vi "CleanUp.vi"(8 "error in (no error)":errorcluster, 11 "Prueba06 in":refnum<class "Prueba06.lvclass">) -> (0 "error out":errorcluster, 3 "Prueba06 out":refnum<class "Prueba06.lvclass">)   [LabVIEW 2019, in "Prueba06.lvclass"]
uses:
  Prueba06.lvclass
  C:/Users/ivan_/Documents/procal/Pruebas/Prueba/Prueba.lvclass
  Prueba/Prueba.lvclass/Prueba.ctl
  Prueba06.lvclass/Prueba06.ctl
  Base de Datos/SQLiteConnector/SQLiteConnection.lvclass
  Base de Datos/Base de Datos.lvclass
  Prueba/Prueba.lvclass
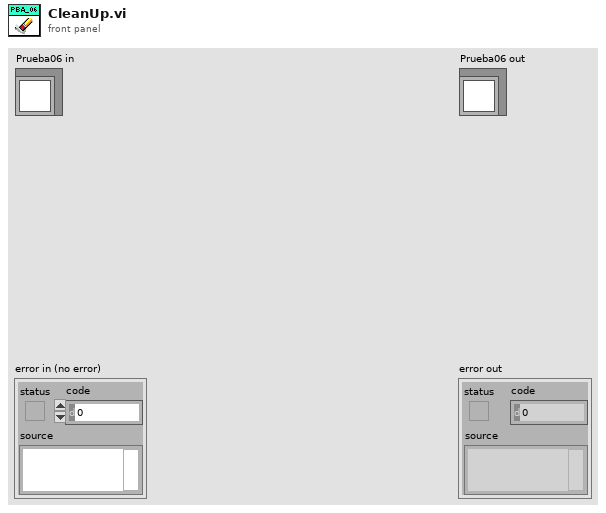
[diagram p1: front panel]
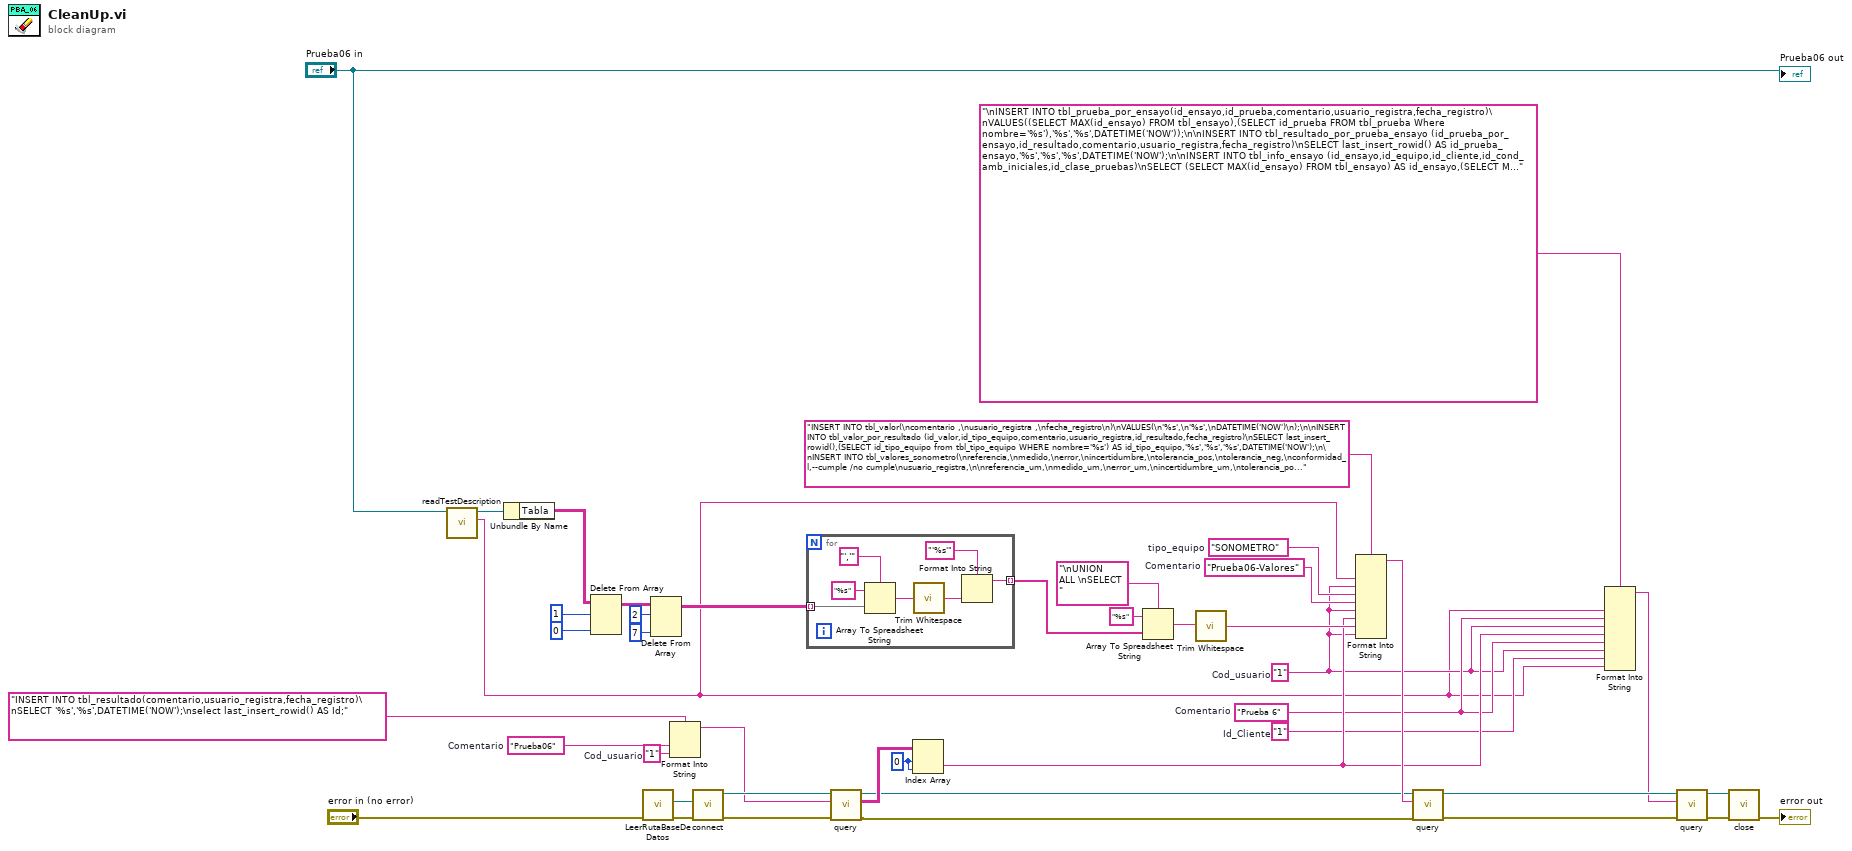
[diagram p0: block diagram]
diagram:
  w15 = "1"  # Id_Cliente
  w16 = "Prueba 6"  # Comentario
  w25 = "SONOMETRO"  # tipo_equipo
  w24 = "Prueba06-Valores"  # Comentario
  w30 = 0 ("index (row)")
  w32 = "1"  # Cod_usuario
  w33 = "Prueba06"  # Comentario
  w14 = "1"  # Cod_usuario
  n1 = call "readTestDescription.vi"("Prueba in"="Prueba06 in") -> ("Test Description"=w4:string, "Prueba out"=w5:refnum<class "Prueba06.lvclass">)  [unwired: 8 in, 1 out]
  n2 = Unbundle By Name(w5) -> ("Tabla"=w8:string[][])
  n3 = Delete From Array(array=w8, length=1, index (col)=0 ("disabled index (col)")) -> (array with subset deleted=w10:string[][])  [unwired: 1 in, 1 out]
  n4 = call "LeerRutaBaseDeDatos.vi"("error in (no error)"="error in (no error)") -> ("error out"=w38:errorcluster, "Database Path"=w37:path)  [unwired: 9 in]
  n5 = Delete From Array(array=w10, length=2, index (col)=7 ("disabled index (col)")) -> (array with subset deleted=w12:string[][])  [unwired: 1 in, 1 out]
  n6 = Format Into String(format string="INSERT INTO tbl_resultado(comentario,usuario_registra,fecha_registro)\nSELECT '%s','%s',DATETIME('NOW');\nselect last_insert_rowid() AS Id;" ("SQL Statement"), w33, w32) -> (resulting string=w31:string)  [unwired: 2 in, 1 out]
  n7 = call "connect.vi"("error in (no error)"=w38, "Database Path"=w37) -> ("error out"=w29:errorcluster, "object out"=w35:refnum<class "SQLiteConnection.lvclass">)  [unwired: 8 in]
  n8 = for {
    tunnel: w12 -> [w44] mode=indexing
    tunnel: [w47] -> w41 mode=indexing
    n9 = Array To Spreadsheet String(delimiter (Tab)="','", array=w44, 3:"%s" ("format string")) -> (spreadsheet string=w46:string)
    n10 = call <vilib>:"Trim Whitespace.vi"("string"=w46) -> ("trimmed string"=w45:string)  [unwired: 1 in]
    n11 = Format Into String(format string="'%s'", w45) -> (resulting string=w47:string)  [unwired: 2 in, 1 out]
  }
  n12 = call "query.vi"("error in (no error)"=w29, "SQL Statement"=w31, "object in"=w35) -> ("error out"=w9:errorcluster, "result"=w28:string[][], "object out"=w27:refnum<class "SQLiteConnection.lvclass">)  [unwired: 5 in, 1 out]
  n13 = Index Array(array=w28, index (row)=w30, index (col)=w30) -> (element=w17:string)
  n14 = Array To Spreadsheet String(delimiter (Tab)="\nUNION ALL \nSELECT ", array=w41, 3:"%s" ("format string")) -> (spreadsheet string=w40:string)
  n15 = call <vilib>:"Trim Whitespace.vi"("string"=w40) -> ("trimmed string"=w26:string)  [unwired: 1 in]
  n16 = Format Into String(format string="INSERT INTO tbl_valor(\ncomentario ,\nusuario_registra ,\nfecha_registro\n)\nVALUES(\n'%s',\n'%s',\nDATETIME('NOW')\n);\n\nINSERT INTO tbl_valor_por_resultado (id_valor,id_tipo_equipo,comentario,usuario_registra,id_resultado,fecha_registro)\nSELECT last_insert_rowid(),(SELECT id_tipo_equipo from tbl_tipo_equipo WHERE nombre='%s') AS id_tipo_equipo,'%s','%s','%s',DATETIME('NOW');\n\nINSERT INTO tbl_valores_sonometro(\nreferencia,\nmedido,\nerror,\nincertidumbre,\ntolerancia_pos,\ntolerancia_neg,\nconformidad_l,--cumple /no cumple\nusuario_registra,\n\nreferencia_um,\nmedido_um,\nerror_um,\nincertidumbre_um,\ntolerancia_pos_um,\ntolerancia_neg_um,\n\nid_valor,\nfecha_registro\n)\nSELECT * FROM(\nSELECT %s\n) AS T\nINNER JOIN\n(SELECT %s AS usuario,'dB','dB','dB','dB','dB','dB',(SELECT MAX(id_valor) FROM tbl_valor) AS id_valor,DATETIME('NOW') fecha ) AS F;\n", w4, w14, w25, w24, w14, w17, w26, w14) -> (resulting string=w36:string)  [unwired: 2 in, 1 out]
  n17 = call "query.vi"("error in (no error)"=w9, "SQL Statement"=w36, "object in"=w27) -> ("error out"=w21:errorcluster, "object out"=w23:refnum<class "SQLiteConnection.lvclass">)  [unwired: 5 in, 2 out]
  n18 = Format Into String(format string="\nINSERT INTO tbl_prueba_por_ensayo(id_ensayo,id_prueba,comentario,usuario_registra,fecha_registro)\nVALUES((SELECT MAX(id_ensayo) FROM tbl_ensayo),(SELECT id_prueba FROM tbl_prueba Where nombre='%s'),'%s','%s',DATETIME('NOW'));\n\nINSERT INTO tbl_resultado_por_prueba_ensayo (id_prueba_por_ensayo,id_resultado,comentario,usuario_registra,fecha_registro)\nSELECT last_insert_rowid() AS id_prueba_ensayo,'%s','%s','%s',DATETIME('NOW');\n\nINSERT INTO tbl_info_ensayo (id_ensayo,id_equipo,id_cliente,id_cond_amb_iniciales,id_clase_pruebas)\nSELECT (SELECT MAX(id_ensayo) FROM tbl_ensayo) AS id_ensayo,(SELECT MAX(id_equipo) FROM tbl_equipo) AS id_equipo,'%s' AS id_cliente,(SELECT MAX(id_cond_amb_iniciales) FROM tbl_cond_amb_iniciales) AS id_cond_amb_iniciales,\n(SELECT id_clase_prueba FROM tbl_clase_prueba WHERE id_clase=(SELECT id_clase FROM tbl_equipo ORDER BY id_equipo DESC LIMIT 1)  AND id_prueba=(SELECT id_prueba FROM tbl_prueba Where nombre='%s')) AS id_clase_pruebas;\n", w4, w16, w14, w17, w16, w14, w15, w4) -> (resulting string=w18:string)  [unwired: 2 in, 1 out]
  n19 = call "query.vi"("error in (no error)"=w21, "SQL Statement"=w18, "object in"=w23) -> ("error out"=w20:errorcluster, "object out"=w22:refnum<class "SQLiteConnection.lvclass">)  [unwired: 5 in, 2 out]
  n20 = call-dynamic "close.vi"("error in (no error)"=w20, "object in"=w22) -> ("error out"=→"error out":errorcluster)  [unwired: 8 in, 1 out]
  "Prueba06 out" <- "Prueba06 in"
